vi "StrToJason.vi"(7 "error in (no error)":errorcluster, 10 "Channel in":refnum<class "Channel.lvclass">) -> (0 "error out":errorcluster, 3 "Channel out":refnum<class "Channel.lvclass">)   [LabVIEW 2018, in "Channel.lvclass"]
uses:
  Channel.lvclass
  Channel.lvclass/Channel.ctl
panel:
  out "JSON":string
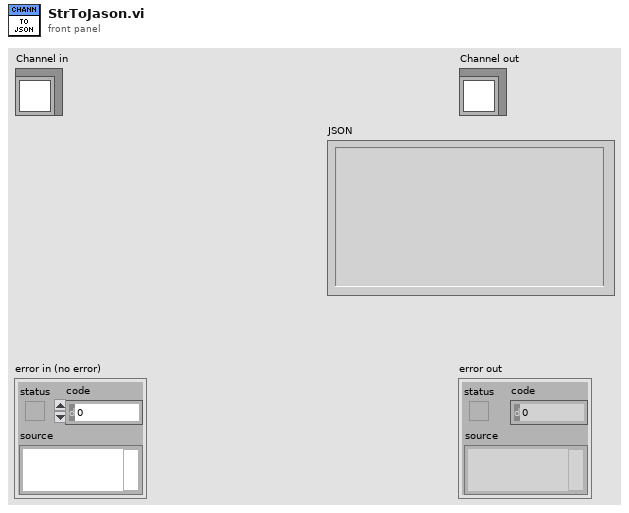
[diagram p1: front panel]
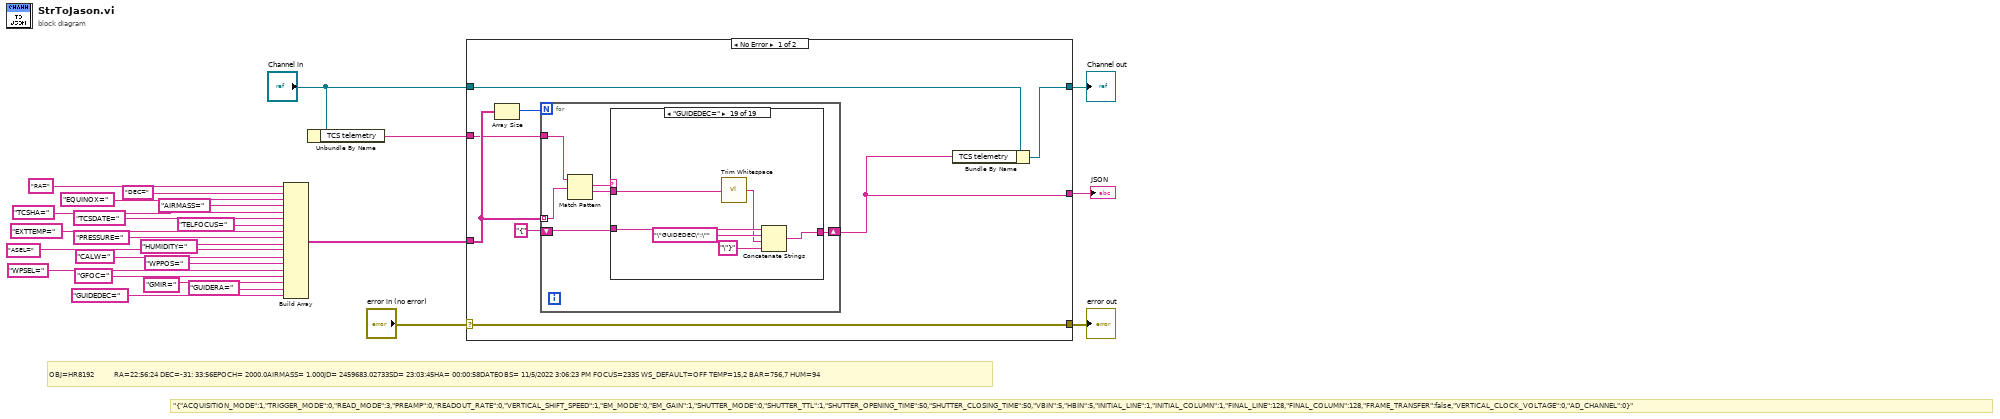
[diagram p0: block diagram]
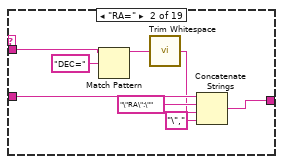
[diagram p3: hidden frame]
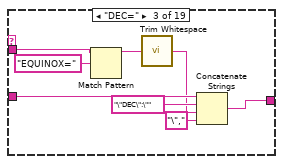
[diagram p4: hidden frame]
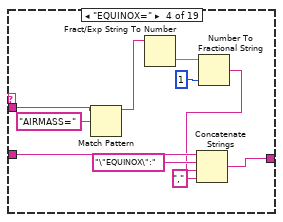
[diagram p5: hidden frame]
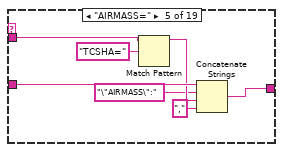
[diagram p6: hidden frame]
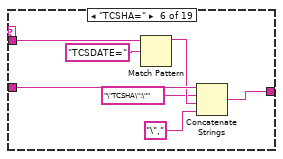
[diagram p7: hidden frame]
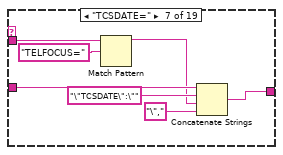
[diagram p8: hidden frame]
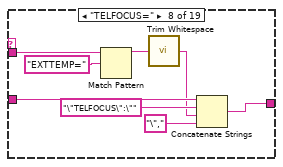
[diagram p9: hidden frame]
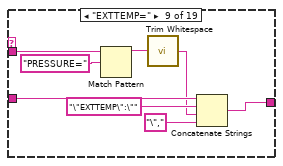
[diagram p10: hidden frame]
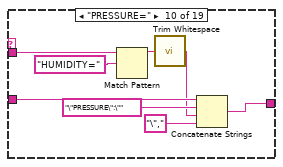
[diagram p11: hidden frame]
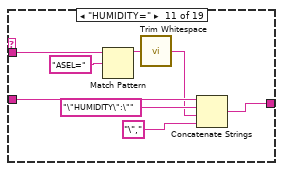
[diagram p12: hidden frame]
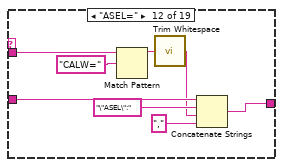
[diagram p13: hidden frame]
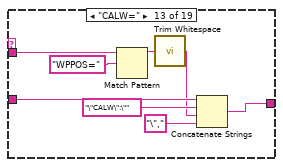
[diagram p14: hidden frame]
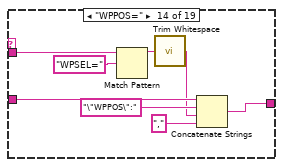
[diagram p15: hidden frame]
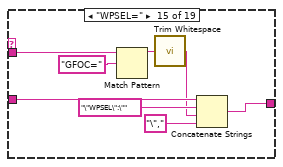
[diagram p16: hidden frame]
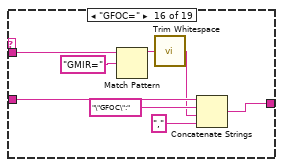
[diagram p17: hidden frame]
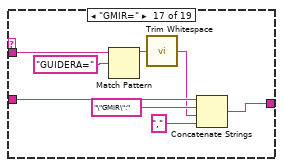
[diagram p18: hidden frame]
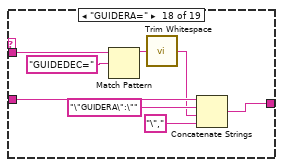
[diagram p19: hidden frame]
diagram:
  # "\"{\"ACQUISITION_MODE\":1,\"TRIGGER_MODE\":0,\"READ_MODE\":3,\"PREAMP\":0,\"READOUT_RATE\":0,\"VERTICAL_SHIFT_SPEED\":1,\"EM_MODE\":0,\"EM_GAIN\":1,\"SHUTTER_MODE\":0,\"SHUTTER_TTL\":1,\"SHUTTER_OPENING_TIME\":50,\"SHUTTER_CLOSING_TIME\":50,\"VBIN\":5,\"HBIN\":5,\"INITIAL_LINE\":1,\"INITIAL_COLUMN\":1,\"FINAL_LINE\":128,\"FINAL_COLUMN\":128,\"FRAME_TRANSFER\":false,\"VERTICAL_CLOCK_VOLTAGE\":0,\"AD_CHANNEL\":0}\""
  # "OBJ=HR8192          RA=22:56:24 DEC=-31: 33:56EPOCH= 2000.0AIRMASS= 1.000JD= 2459683.02733SD= 23:03:45HA= 00:00:58DATEOBS= 11/5/2022 3:06:23 PM FOCUS=233S WS_DEFAULT=OFF TEMP=15,2 BAR=756,7 HUM=94"
  n1 = Build Array("RA=", "DEC=", "EQUINOX=", "AIRMASS=", "TCSHA=", "TCSDATE=", "TELFOCUS=", "EXTTEMP=", "PRESSURE=", "HUMIDITY=", "ASEL=", "CALW=", "WPPOS=", "WPSEL=", "GFOC=", "GMIR=", "GUIDERA=", "GUIDEDEC=") -> (w11:string[])
  n2 = Unbundle By Name("Channel in") -> ("TCS telemetry"=w9:string)
  n3 = case shown="No Error" "error in (no error)" {
    selector: "error in (no error)" -> [w33 w184]
    tunnel: [w33 w184] -> w24
    tunnel: [w28 w183] -> w23
    tunnel: "Channel in" -> [w29 w183]
    tunnel: [w27 w182] -> w22
    tunnel: w9 -> [w26 w182]
    tunnel: w11 -> [w32 _]
    frame No Error {
      n4 = Array Size(array=w32) -> (size(s)=w31:i32)
      n5 = for {
        N: w31 -> [_]
        tunnel: w32 -> [w39] mode=indexing
        shift-right: [w35] -> w27
        shift-left: "{" -> [w36]
        tunnel: w26 -> [w34]
        n6 = Match Pattern(string=w34, regular expression=w39) -> (match substring=w38:string, after substring=w37:string)  [unwired: 1 in, 2 out]
        n7 = case shown="\"GUIDEDEC=\"" w38 {
          tunnel: w37 -> [_ w47 w55 w65 w72 w79 w86 w94 w102 w110 w113 w126 w134 w142 w150 w158 w161 w169 w176]
          tunnel: w36 -> [w40 w46 w54 w64 w71 w78 w85 w93 w101 w109 w119 w125 w133 w141 w149 w157 w167 w175 w181]
          tunnel: [w40 w45 w53 w63 w70 w77 w84 w92 w100 w108 w118 w124 w132 w140 w148 w156 w166 w174 w180] -> w35
          frame Default {
          }
          frame "RA=" {
            n8 = Match Pattern(string=w47, regular expression="DEC=") -> (before substring=w44:string)  [unwired: 1 in, 3 out]
            n9 = call <vilib>:"Trim Whitespace.vi"("string"=w44) -> ("trimmed string"=w41:string)  [unwired: 1 in]
            n10 = Concatenate Strings(w46, "\"RA\":\"" ("string"), w41, "\"," ("string")) -> (w45:string)
          }
          frame "DEC=" {
            n11 = Match Pattern(string=w55, regular expression="EQUINOX=") -> (before substring=w52:string)  [unwired: 1 in, 3 out]
            n12 = call <vilib>:"Trim Whitespace.vi"("string"=w52) -> ("trimmed string"=w49:string)  [unwired: 1 in]
            n13 = Concatenate Strings(w54, "\"DEC\":\"" ("string"), w49, "\"," ("string")) -> (w53:string)
          }
          frame "EQUINOX=" {
            n14 = Match Pattern(string=w65, regular expression="AIRMASS=") -> (before substring=w60:string)  [unwired: 1 in, 3 out]
            n15 = Fract/Exp String To Number(string=w60) -> (number=w59:dbl)  [unwired: 3 in, 1 out]
            n16 = Number To Fractional String(number=w59, precision (6)=i16 1) -> (F-format string=w58:string)  [unwired: 2 in]
            n17 = Concatenate Strings(w64, "\"EQUINOX\":" ("string"), w58, "," ("string")) -> (w63:string)
          }
          frame "AIRMASS=" {
            n18 = Match Pattern(string=w72, regular expression="TCSHA=") -> (before substring=w69:string)  [unwired: 1 in, 3 out]
            n19 = Concatenate Strings(w71, "\"AIRMASS\":" ("string"), w69, "," ("string")) -> (w70:string)
          }
          frame "TCSHA=" {
            n20 = Match Pattern(string=w79, regular expression="TCSDATE=") -> (before substring=w76:string)  [unwired: 1 in, 3 out]
            n21 = Concatenate Strings(w78, "\"TCSHA\":\"" ("string"), w76, "\"," ("string")) -> (w77:string)
          }
          frame "TCSDATE=" {
            n22 = Match Pattern(string=w86, regular expression="TELFOCUS=") -> (before substring=w81:string)  [unwired: 1 in, 3 out]
            n23 = Concatenate Strings(w85, "\"TCSDATE\":\"" ("string"), w81, "\"," ("string")) -> (w84:string)
          }
          frame "TELFOCUS=" {
            n24 = Match Pattern(string=w94, regular expression="EXTTEMP=") -> (before substring=w91:string)  [unwired: 1 in, 3 out]
            n25 = call <vilib>:"Trim Whitespace.vi"("string"=w91) -> ("trimmed string"=w88:string)  [unwired: 1 in]
            n26 = Concatenate Strings(w93, "\"TELFOCUS\":\"" ("string"), w88, "\"," ("string")) -> (w92:string)
          }
          frame "EXTTEMP=" {
            n27 = Match Pattern(string=w102, regular expression="PRESSURE=") -> (before substring=w97:string)  [unwired: 1 in, 3 out]
            n28 = call <vilib>:"Trim Whitespace.vi"("string"=w97) -> ("trimmed string"=w96:string)  [unwired: 1 in]
            n29 = Concatenate Strings(w101, "\"EXTTEMP\":\"" ("string"), w96, "\"," ("string")) -> (w100:string)
          }
          frame "PRESSURE=" {
            n30 = Match Pattern(string=w110, regular expression="HUMIDITY=") -> (before substring=w107:string)  [unwired: 1 in, 3 out]
            n31 = call <vilib>:"Trim Whitespace.vi"("string"=w107) -> ("trimmed string"=w104:string)  [unwired: 1 in]
            n32 = Concatenate Strings(w109, "\"PRESSURE\":\"" ("string"), w104, "\"," ("string")) -> (w108:string)
          }
          frame "HUMIDITY=" {
            n33 = Match Pattern(string=w113, regular expression="ASEL=") -> (before substring=w114:string)  [unwired: 1 in, 3 out]
            n34 = call <vilib>:"Trim Whitespace.vi"("string"=w114) -> ("trimmed string"=w112:string)  [unwired: 1 in]
            n35 = Concatenate Strings(w119, "\"HUMIDITY\":\"" ("string"), w112, "\"," ("string")) -> (w118:string)
          }
          frame "ASEL=" {
            n36 = Match Pattern(string=w126, regular expression="CALW=") -> (before substring=w123:string)  [unwired: 1 in, 3 out]
            n37 = call <vilib>:"Trim Whitespace.vi"("string"=w123) -> ("trimmed string"=w120:string)  [unwired: 1 in]
            n38 = Concatenate Strings(w125, "\"ASEL\":" ("string"), w120, "," ("string")) -> (w124:string)
          }
          frame "CALW=" {
            n39 = Match Pattern(string=w134, regular expression="WPPOS=") -> (before substring=w131:string)  [unwired: 1 in, 3 out]
            n40 = call <vilib>:"Trim Whitespace.vi"("string"=w131) -> ("trimmed string"=w128:string)  [unwired: 1 in]
            n41 = Concatenate Strings(w133, "\"CALW\":\"" ("string"), w128, "\"," ("string")) -> (w132:string)
          }
          frame "WPPOS=" {
            n42 = Match Pattern(string=w142, regular expression="WPSEL=") -> (before substring=w139:string)  [unwired: 1 in, 3 out]
            n43 = call <vilib>:"Trim Whitespace.vi"("string"=w139) -> ("trimmed string"=w136:string)  [unwired: 1 in]
            n44 = Concatenate Strings(w141, "\"WPPOS\":" ("string"), w136, "," ("string")) -> (w140:string)
          }
          frame "WPSEL=" {
            n45 = Match Pattern(string=w150, regular expression="GFOC=") -> (before substring=w147:string)  [unwired: 1 in, 3 out]
            n46 = call <vilib>:"Trim Whitespace.vi"("string"=w147) -> ("trimmed string"=w144:string)  [unwired: 1 in]
            n47 = Concatenate Strings(w149, "\"WPSEL\":\"" ("string"), w144, "\"," ("string")) -> (w148:string)
          }
          frame "GFOC=" {
            n48 = Match Pattern(string=w158, regular expression="GMIR=") -> (before substring=w155:string)  [unwired: 1 in, 3 out]
            n49 = call <vilib>:"Trim Whitespace.vi"("string"=w155) -> ("trimmed string"=w152:string)  [unwired: 1 in]
            n50 = Concatenate Strings(w157, "\"GFOC\":" ("string"), w152, "," ("string")) -> (w156:string)
          }
          frame "GMIR=" {
            n51 = Match Pattern(string=w161, regular expression="GUIDERA=") -> (before substring=w162:string)  [unwired: 1 in, 3 out]
            n52 = call <vilib>:"Trim Whitespace.vi"("string"=w162) -> ("trimmed string"=w160:string)  [unwired: 1 in]
            n53 = Concatenate Strings(w167, "\"GMIR\":" ("string"), w160, "," ("string")) -> (w166:string)
          }
          frame "GUIDERA=" {
            n54 = Match Pattern(string=w169, regular expression="GUIDEDEC=") -> (before substring=w170:string)  [unwired: 1 in, 3 out]
            n55 = call <vilib>:"Trim Whitespace.vi"("string"=w170) -> ("trimmed string"=w168:string)  [unwired: 1 in]
            n56 = Concatenate Strings(w175, "\"GUIDERA\":\"" ("string"), w168, "\"," ("string")) -> (w174:string)
          }
          frame "GUIDEDEC=" {
            n57 = call <vilib>:"Trim Whitespace.vi"("string"=w176) -> ("trimmed string"=w177:string)  [unwired: 1 in]
            n58 = Concatenate Strings(w181, "\"GUIDEDEC\":\"" ("string"), w177, "\"}" ("string")) -> (w180:string)
          }
        }
      }
      n59 = Bundle By Name(cluster=w29, "TCS telemetry"=w27) -> (w28:refnum<class "Channel.lvclass">)
    }
    frame Error {
    }
  }
  "error out" <- w24
  "Channel out" <- w23
  "JSON" <- w22
